vi "Abort.vi"(8 "error in (no error)":errorcluster, 11 "AbortsAPI in":refnum<class "AbortAPI.lvclass">) -> (0 "error out":errorcluster, 3 "AbortsAPI out":refnum<class "AbortAPI.lvclass">)   [LabVIEW 2020, in "Volatus.lvlib" / "AbortAPI.lvclass"]
uses:
  AbortAPI.lvclass
  AbortAPI.lvclass/AbortAPI.ctl
  AbortHandler Messages/Abort Msg/Abort Msg.lvclass
  <vilib>/ActorFramework/Message Enqueuer/Message Priority.ctl
  <vilib>/ActorFramework/Message Enqueuer/Message Enqueuer.lvclass
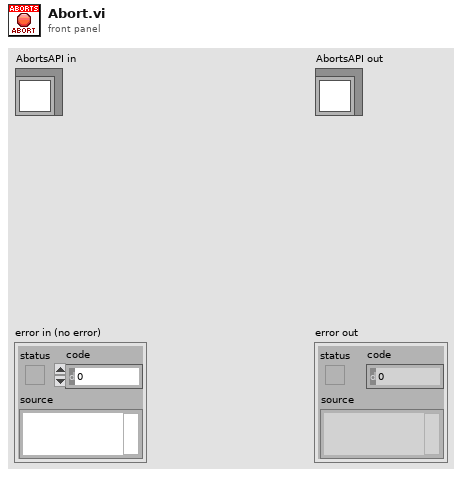
[diagram p1: front panel]
types:
  T1 = typedef "Actor Framework.lvlib/Message Enqueuer.lvclass/Message Priority.ctl" = enum16{"Low", "Normal", "High"}
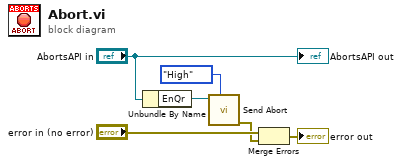
[diagram p0: block diagram]
diagram:
  n1 = Unbundle By Name("AbortsAPI in") -> ("EnQr"=w4:refnum<class "Message Enqueuer.lvclass">)
  n2 = call "Send Abort.vi"("Message Priority (Normal)"=Message_Priority."High", "Message Enqueuer"=w4) -> ("error out"=w2:errorcluster)  [unwired: 8 in, 1 out]
  n3 = Merge Errors("error in (no error)", w2) -> (→"error out":errorcluster)
  "AbortsAPI out" <- "AbortsAPI in"
